vi "OSC_Read.vi"(0 "instrument handle In":refnum<k15>, 1 "string":string="RES", 2 "appended path In":path, 3 "file path (dialog if empty)":path=path "D:/GSSor/Test_OSC/LOGS", 5 "error IO In":errorcluster, 7 "channel name":string="0" caption="Channel Name(s)", 9 "timeout (s)":dbl=-1.0 caption="Timeout(s)" format="%.2f", 11 "IterIn":u64=1) -> (4 "instrument handle Out":refnum<k15>, 6 "error IO Out":errorcluster, 8 "Waveform Graph":waveform(dbl)[](graph), 10 "appended path Out":path, 15 "IterOut":u64)   [LabVIEW 2010]
uses:
  <instrlib>/niScope/Controls/niScope timestamp type.ctl
  <vilib>/Waveform/WDTFileIO.llb/Export Waveforms To Spreadsheet File (1D).vi
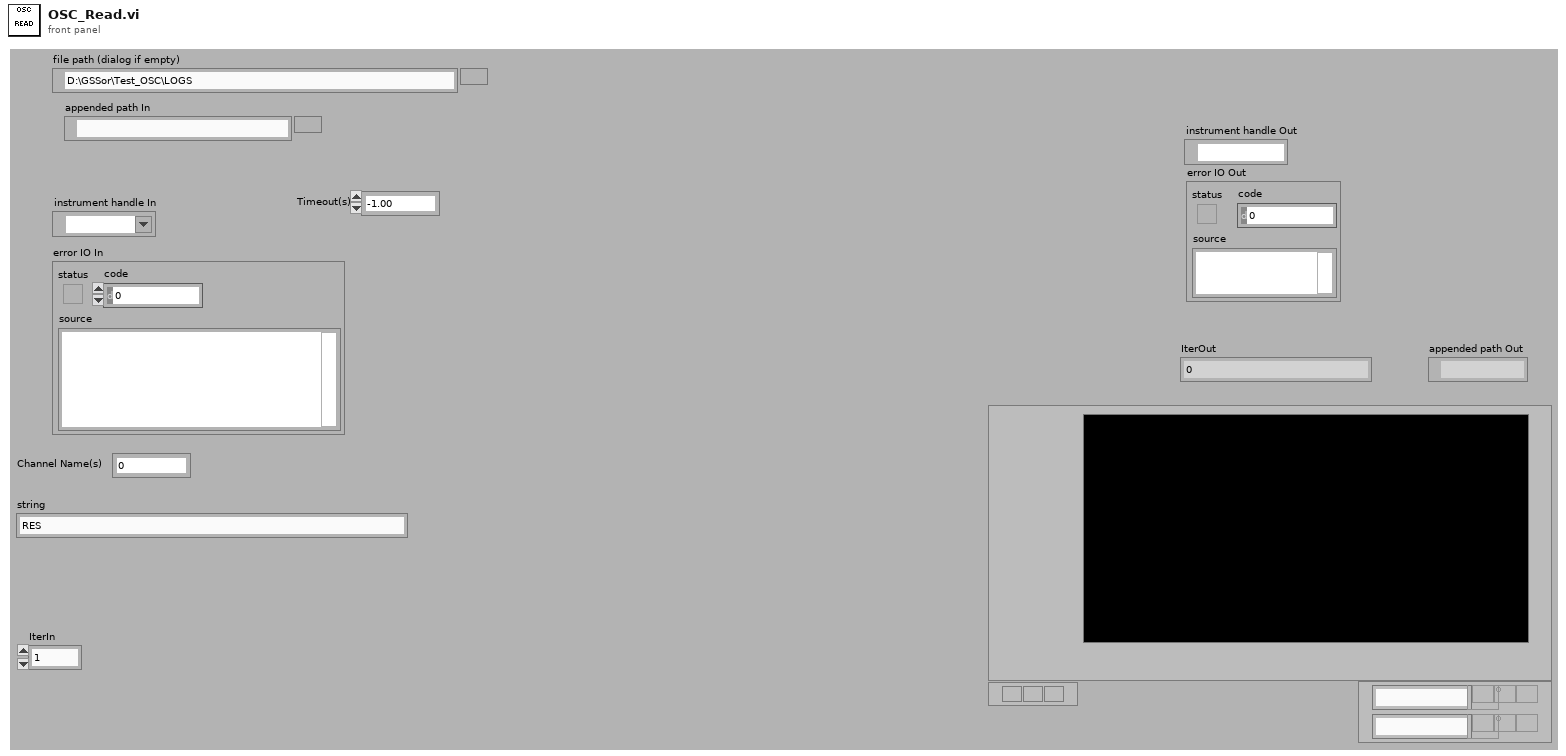
[diagram p1: front panel]
types:
  T1 = typedef "niScope timestamp type.ctl" = i32
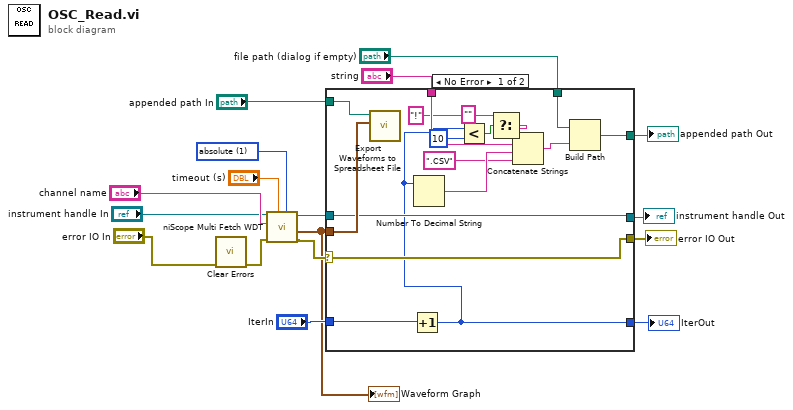
[diagram p0: block diagram]
diagram:
  w5 = T1 1 items=["relative", "absolute"] ("timestamp Type")
  n1 = call <vilib>:"Clear Errors.vi"("error in (no error)"="error IO In") -> ("error out"=w4:errorcluster)  [unwired: 6 in]
  n2 = call "niScope Multi Fetch WDT.vi"("timestamp Type"=w5, "timeout"="timeout (s)", "error in"=w4, "channels"="channel name", "instrument handle"="instrument handle In") -> ("error out"=w8:errorcluster, "wfm"=w3:waveform(dbl)[], "instrument handle out"=w7:refnum<k15>)  [unwired: 3 in, 1 out]
  "Waveform Graph" <- w3
  n3 = case shown="No Error" w8 {
    selector: w8 -> [w27 w35]
    tunnel: "appended path In" -> [w34 w38]
    tunnel: w3 -> [w33 _]
    tunnel: "file path (dialog if empty)" -> [w32 _]
    tunnel: "string" -> [w31 _]
    tunnel: "IterIn" -> [w19 w37]
    tunnel: [w18 w37] -> w14
    tunnel: [w28 w38] -> w16
    tunnel: w7 -> [w26 w36]
    tunnel: [w26 w36] -> w15
    tunnel: [w27 w35] -> w13
    frame No Error {
      n4 = call-poly <vilib>:"Export Waveforms to Spreadsheet File.vi"("waveforms"=w33, "file path (dialog if empty)"=w34) -> ()  [unwired: 8 in, 2 out]
      n5 = Increment(x=w19) -> (x+1=w18:u64)
      n6 = Number To Decimal String(number=w18) -> (decimal integer string=w30:string)  [unwired: 1 in]
      n7 = Less?(x=w18, y=10) -> (x < y?=w23:bool)
      n8 = Select(t="!" ("string"), s=w23, f="") -> (s? t:f=w21:string)
      n9 = Concatenate Strings(w21, w31, w30, ".CSV" ("string")) -> (w29:string)
      n10 = Build Path(base path=w32, name or relative path=w29) -> (appended path=w28:path)
    }
    frame Error {
    }
  }
  "appended path Out" <- w16
  "instrument handle Out" <- w15
  "IterOut" <- w14
  "error IO Out" <- w13
